vi "Draw Label.vi"(4 "Value Color":u32(colorbox)=32639, 6 "Type Color":u32(colorbox)=32639, 7 "Position":T1={"top"=20, "Frame Border"={"left"=0, "top"=0, "right"=150, "bottom"=100}}, 9 "Value":string, 10 "Name":string, 11 "Picture In":picture) -> (3 "Picture":picture)   [LabVIEW 2022 SP3, in "FlexBlocks Support.lvlib"]
uses:
  FlexBlocks Support.lvlib
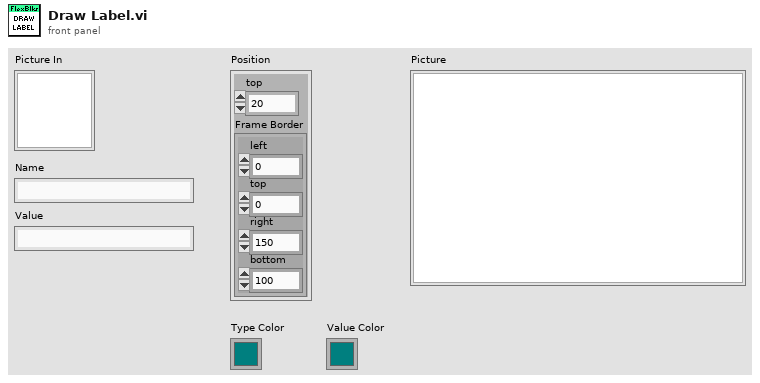
[diagram p1: front panel]
types:
  T1 = cluster{"top":i16, "Frame Border":cluster{"left":i16, "top":i16, "right":i16, "bottom":i16}}
  T2 = cluster{"left":i16, "top":i16, "right":i16, "bottom":i16}
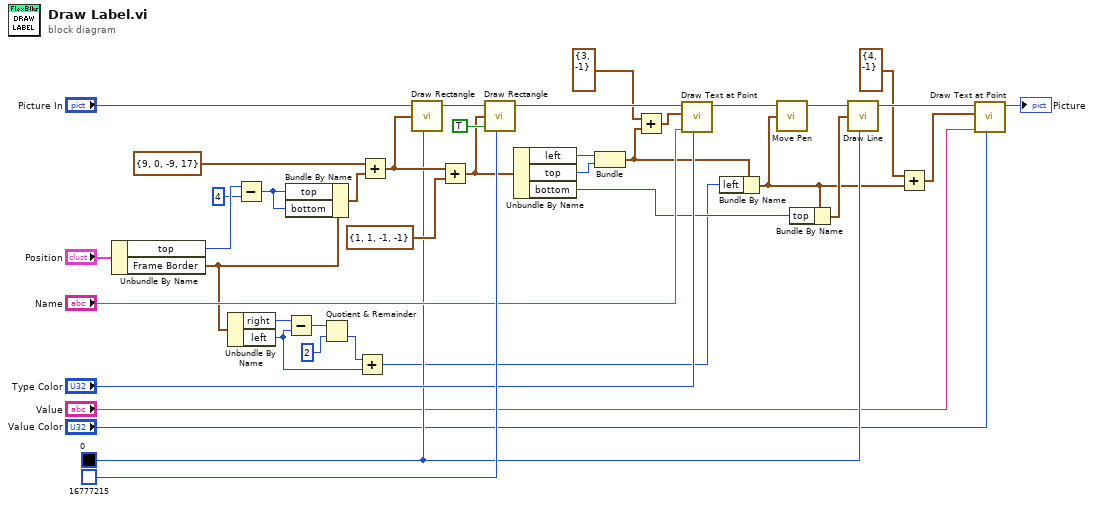
[diagram p0: block diagram]
diagram:
  w14 = u32 0
  n1 = Unbundle By Name("Position") -> ("top"=w38:i16, "Frame Border"=w21:T2)
  n2 = Unbundle By Name(w21) -> ("right"=w20:i16, "left"=w10:i16)
  n3 = Subtract(x=w38, y=i16 4) -> (x-y=w35:i16)
  n4 = Bundle By Name(cluster=w21, "top"=w35, "bottom"=w35) -> (w36:T2)
  n5 = Subtract(x=w20, y=w10) -> (x-y=w19:i16)
  n6 = Quotient & Remainder(x=w19, y=i16 2) -> (floor(x/y)=w11:i16)  [unwired: 1 out]
  n7 = Add(x=w11, y=w10) -> (x+y=w9:i16)
  n8 = Add(x=T2 {"left"=9, "top"=0, "right"=-9, "bottom"=17} ("Frame Border"), y=w36) -> (x+y=w31:T2)
  n9 = call <vilib>:"Draw Rectangle.vi"("picture"="Picture In", "rect"=w31, "color(black)"=w14) -> ("new picture"=w33:picture)  [unwired: 6 in]
  n10 = Add(x=w31, y=T2 {"left"=1, "top"=1, "right"=-1, "bottom"=-1} ("Frame Border")) -> (x+y=w27:T2)
  n11 = call <vilib>:"Draw Rectangle.vi"("picture"=w33, "rect"=w27, "fill?(F)"=TRUE, "color(black)"=u32 16777215) -> ("new picture"=w28:picture)  [unwired: 5 in]
  n12 = Unbundle By Name(w27) -> ("left"=w26:i16, "top"=w25:i16, "bottom"=w13:i16)
  n13 = Bundle("left"=w26, "top"=w25) -> (w15:cluster{"left":i16, "top":i16})  [unwired: 1 in]
  n14 = Add(x=cluster{"left":i16, "top":i16} {"left"=3, "top"=-1} ("output cluster"), y=w15) -> (x+y=w22:cluster{"left":i16, "top":i16})
  n15 = call <vilib>:"Draw Text at Point.vi"("text color(black)"="Type Color", "text"="Name", "origin"=w22, "picture"=w28) -> ("new picture"=w17:picture)  [unwired: 6 in, 1 out]
  n16 = Bundle By Name(cluster=w15, "left"=w9) -> (w7:cluster{"left":i16, "top":i16})
  n17 = call <vilib>:"Move Pen.vi"("new position"=w7, "picture"=w17) -> ("new picture"=w16:picture)  [unwired: 3 in]
  n18 = Bundle By Name(cluster=w7, "top"=w13) -> (w12:cluster{"left":i16, "top":i16})
  n19 = call <vilib>:"Draw Line.vi"("picture"=w16, "end point"=w12, "color(black)"=w14) -> ("new picture"=w8:picture)  [unwired: 6 in]
  n20 = Add(x=cluster{"left":i16, "top":i16} {"left"=4, "top"=-1} ("output cluster"), y=w7) -> (x+y=w5:cluster{"left":i16, "top":i16})
  n21 = call <vilib>:"Draw Text at Point.vi"("text color(black)"="Value Color", "text"="Value", "origin"=w5, "picture"=w8) -> ("new picture"=→"Picture":picture)  [unwired: 6 in, 1 out]
